vi "Parse SHOW STATUS.vi"(8 "error in":errorcluster, 10 "read buffer":string) -> (0 "error out":errorcluster)   [LabVIEW 2019, in "AH2500.lvlib"]
uses:
  AH2500.lvlib
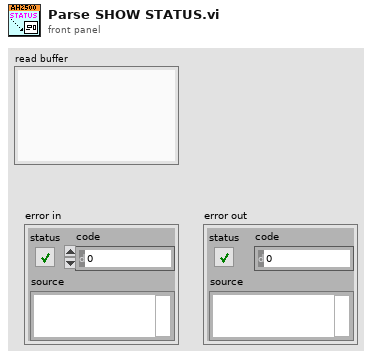
[diagram p1: front panel]
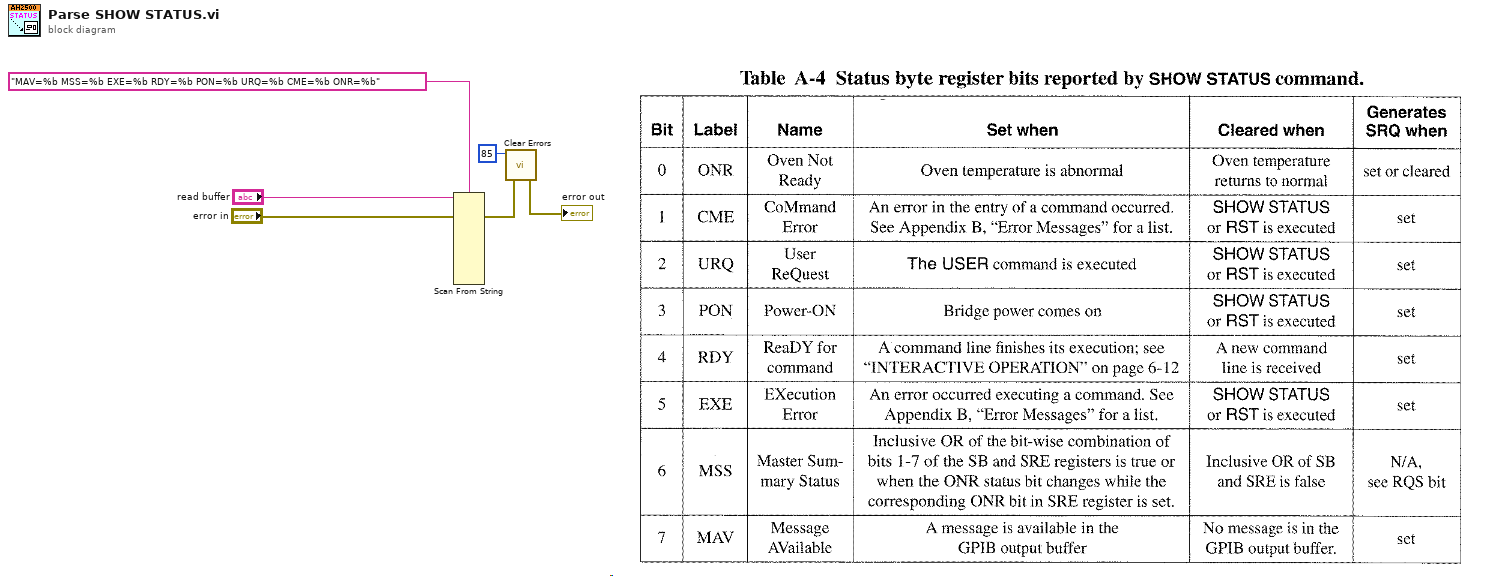
[diagram p0: block diagram]
diagram:
  n1 = Scan From String(format string="MAV=%b MSS=%b EXE=%b RDY=%b PON=%b URQ=%b CME=%b ONR=%b", input string="read buffer", error in="error in") -> (error out=w4:errorcluster)  [unwired: 17 in, 2 out]
  n2 = call <vilib>:"Clear Errors.vi"("error in (no error)"=w4, "specific error code to clear (0: all)"=85) -> ("error out"=→"error out":errorcluster)  [unwired: 4 in, 1 out]
